vi "RT Close  FAST.vi"(1 "error in (no error)":errorcluster) -> (0 "error out":errorcluster)   [LabVIEW 2012]
uses:
  FAST_RT_DLL.dll
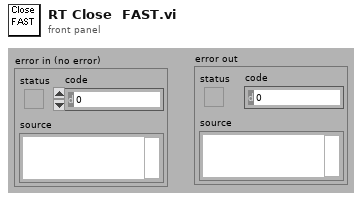
[diagram p1: front panel]
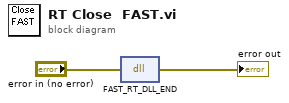
[diagram p0: block diagram]
diagram:
  n1 = dll-call lib="C:/Users/MMonroe/Desktop/Current Opps/FAST RT DLL/demoVI_V8/FAST_RT_DLL.dll" fn="FAST_RT_DLL_END"(error in="error in (no error)") -> (error out=→"error out":errorcluster)  [unwired: 2 in, 2 out]
